vi "ping.vi"(8 "error in (no error)":errorcluster, 11 "Analyze Actor in":refnum<class "Analyze Actor.lvclass">) -> (0 "error out":errorcluster, 3 "Analyze Actor out":refnum<class "Analyze Actor.lvclass">)   [LabVIEW 2014, in "Analyze Actor.lvlib" / "Analyze Actor.lvclass"]
uses:
  Analyze Actor.lvclass
panel:
  # "Ne dozhdjetes!"
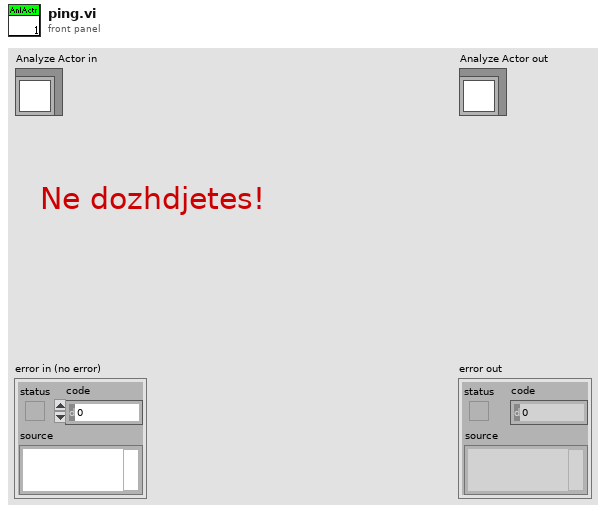
[diagram p1: front panel]
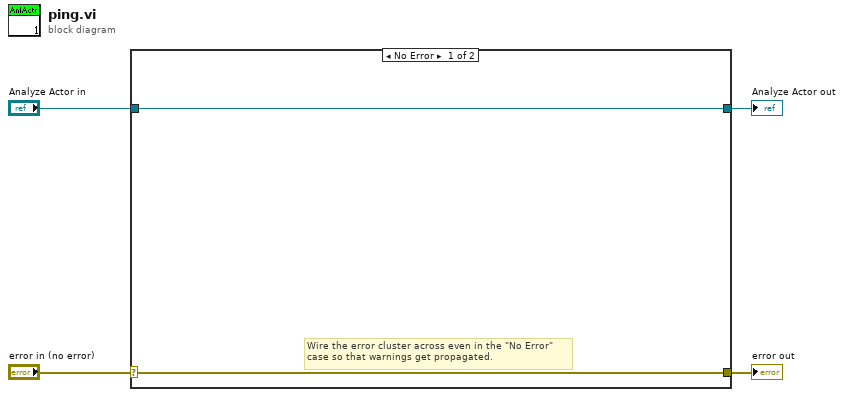
[diagram p0: block diagram]
diagram:
  n1 = case shown="No Error" "error in (no error)" {
    selector: "error in (no error)" -> [w5 w8]
    tunnel: [w5 w8] -> w3
    tunnel: [w6 w7] -> w1
    tunnel: "Analyze Actor in" -> [w6 w7]
    frame No Error {
      # "Wire the error cluster across even in the \"No Error\"\ncase so that warnings get propagated."
    }
    frame Error {
    }
  }
  "error out" <- w3
  "Analyze Actor out" <- w1
